vi "Close Hardware.vi"(8 "error in (no error)":errorcluster, 11 "Instrument in":refnum<class "Instrument.lvclass">) -> (0 "error out":errorcluster, 3 "Instrument out":refnum<class "Instrument.lvclass">)   [LabVIEW 2019, in "Instrument.lvclass"]
doc: "Override to <b>close</b> the connection to your hardware"
uses:
  Instrument.lvclass
  subsystems/HAL/HAL.lvclass
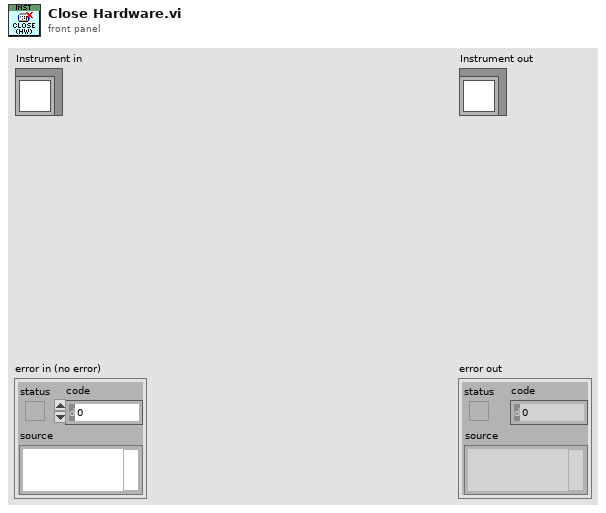
[diagram p1: front panel]
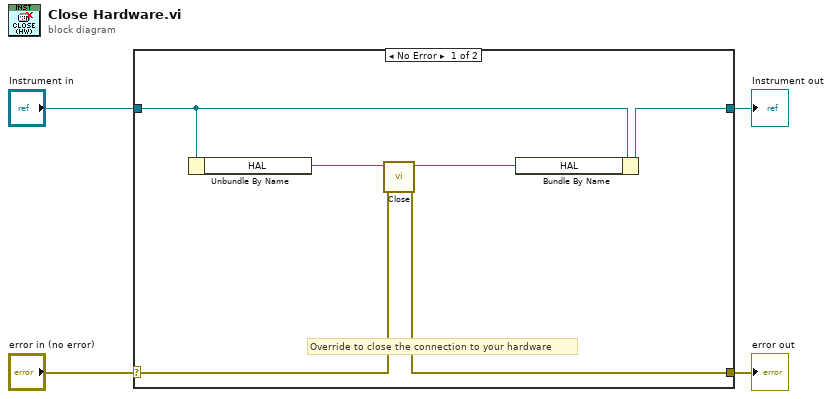
[diagram p0: block diagram]
diagram:
  n1 = case shown="No Error" "error in (no error)" {
    selector: "error in (no error)" -> [w8 w12]
    tunnel: [w7 w12] -> w3
    tunnel: [w6 w11] -> w1
    tunnel: "Instrument in" -> [w5 w11]
    frame No Error {
      # "Override to close the connection to your hardware"
      n2 = Unbundle By Name(w5) -> ("HAL"=w10:refnum<class "HAL.lvclass">)
      n3 = call-dynamic "Close.vi"("error in (no error)"=w8, "HAL in"=w10) -> ("error out"=w7:errorcluster, "HAL out"=w9:refnum<class "HAL.lvclass">)  [unwired: 8 in]
      n4 = Bundle By Name(cluster=w5, "HAL"=w9) -> (w6:refnum<class "Instrument.lvclass">)
    }
    frame Error {
    }
  }
  "error out" <- w3
  "Instrument out" <- w1
